vi "Write Attribute.vi"(4 "Attribute":variant, 6 "Attribute Name":string, 11 "Executioner in":refnum<class "Executioner.lvclass">) -> (3 "Executioner out":refnum<class "Executioner.lvclass">)   [LabVIEW 2017, in "Test Executive.lvlib" / "Executioner.lvclass"]
uses:
  <vilib>/gpm_packages/@cs/test-executive/Source/Test Executive/Executioner/Executioner.lvclass
  <vilib>/gpm_packages/@cs/test-executive/Source/Test Executive/Executioner/Executioner.lvclass/Executioner.ctl
  <vilib>/gpm_packages/@cs/lookup-table/Source/LookupTable/LookupTable.lvclass/LookupTable.ctl
  34a0310f-deee-4535-ad7a-b3ba66525344.vi
  <vilib>/gpm_packages/@cs/lookup-table/Source/LookupTable/Read Table Reference.vi
  34a0310f-deee-4535-ad7a-b3ba66525344.vi/32bef235-b709-4b03-b4cf-645855fba0ce.vi
  <vilib>/gpm_packages/@cs/lookup-table/Source/LookupTable/LookupTable.lvclass
panel:
  out "error out":errorcluster
  out "Replaced?":bool
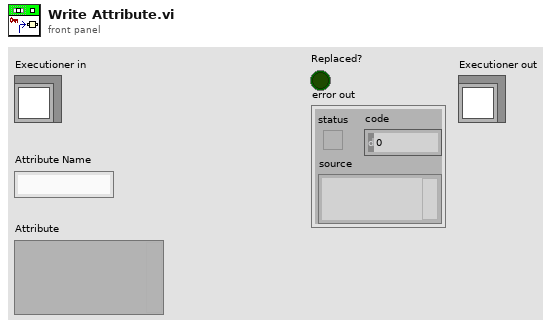
[diagram p1: front panel]
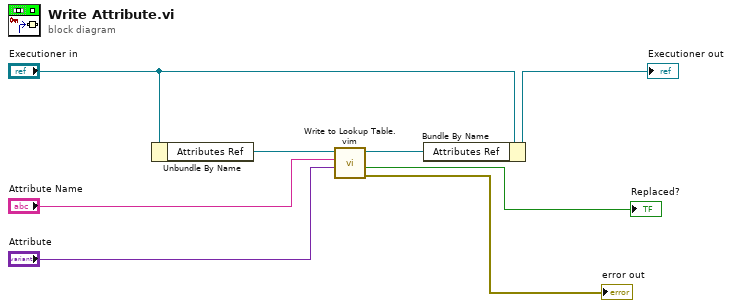
[diagram p0: block diagram]
diagram:
  n1 = Unbundle By Name("Executioner in") -> ("Attributes Ref"=w8:refnum<data-value>)
  n2 = call "Write to Lookup Table.vim"("Item"="Attribute", "Item Name"="Attribute Name", "LookupTable Reference"=w8) -> ("error out"=→"error out":errorcluster, "Replaced?"=→"Replaced?":bool, "LookupTable Reference Out"=w1:refnum<data-value>)  [unwired: 6 in]
  n3 = Bundle By Name(cluster="Executioner in", "Attributes Ref"=w1) -> (→"Executioner out":refnum<class "Executioner.lvclass">)
